vi "Event Loop Async.vi"(8 "error in (no error)":errorcluster, 11 "PanelArray in":refnum<class "PanelArray.lvclass">) -> ()   [LabVIEW 2018, in "OOPanel.lvlib" / "PanelArray.lvclass"]
uses:
  PanelArray.lvclass
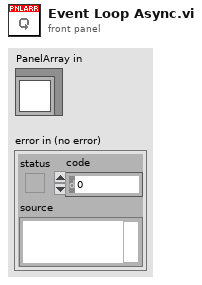
[diagram p1: front panel]
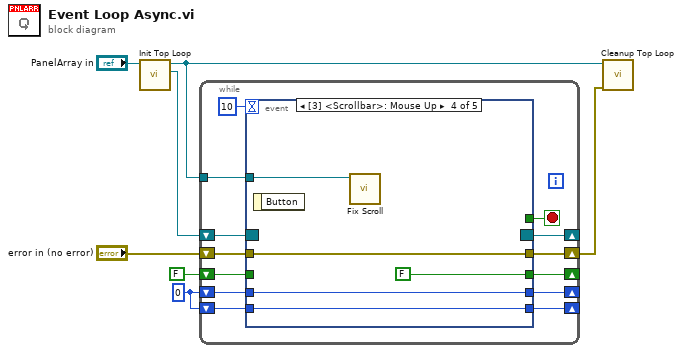
[diagram p0: block diagram]
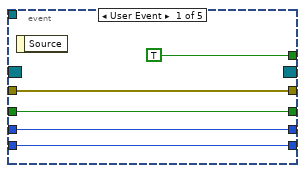
[diagram p2: hidden frame]
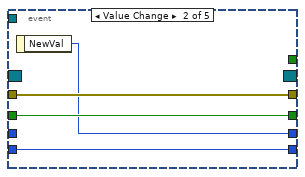
[diagram p3: hidden frame]
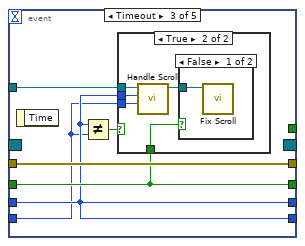
[diagram p4: hidden frame]
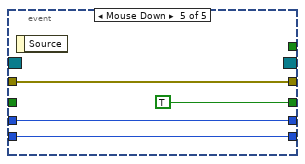
[diagram p7: hidden frame]
diagram:
  w1 = 0
  n1 = call "Init Top Loop.vi"("PanelArray in"="PanelArray in") -> ("Event Registration Refnum"=w6:refnum<event-registration>, "PanelArray out"=w4:refnum<class "PanelArray.lvclass">)  [unwired: 8 in, 1 out]
  n2 = while {
    tunnel: w4 -> [w19]
    shift-right: [w18] -> _
    shift-left: w6 -> [w20]
    shift-right: [w15] -> w3
    shift-left: "error in (no error)" -> [w16]
    shift-right: [w13] -> _
    shift-left: FALSE -> [w14]
    shift-right: [w9] -> _
    shift-left: w1 -> [w11]
    shift-right: [w8] -> _
    shift-left: w1 -> [w10]
    stop <- w17 stop-if-true
    n3 = event shown="[3] <Scrollbar>: Mouse Up" {
      selector: w20 -> [_ _ _ _ _]
      dyn-events: [_ _ _ _ _] -> w18
      timeout: 10 -> [_ _ _ _ _]
      tunnel: w19 -> [_ _ w34 w42 _]
      tunnel: [TRUE _ _ _ _] -> w17
      tunnel: w16 -> [w24 w29 w35 w46 w50]
      tunnel: [w24 w29 w35 w46 w50] -> w15
      tunnel: w14 -> [w23 w28 w33 _ _]
      tunnel: [w23 w28 w33 FALSE TRUE] -> w13
      tunnel: w11 -> [w21 _ w32 w43 w47]
      tunnel: w10 -> [w22 w26 w31 w44 w48]
      tunnel: [w21 w27 w32 w43 w47] -> w9
      tunnel: [w22 w26 w32 w44 w48] -> w8
      event User Event {
        n4 = event-data() -> ()  [unwired: 1 in, 1 out]
      }
      event Value Change {
        n5 = event-data() -> ("NewVal"=w27:i32)  [unwired: 1 in]
      }
      event Timeout {
        n6 = event-data() -> ()  [unwired: 1 in, 1 out]
        n7 = Not Equal?(x=w32, y=w31) -> (x != y?=w30:bool)
        n8 = case shown="True" w30 {
          tunnel: w34 -> [_ w40]
          tunnel: w32 -> [_ w39]
          tunnel: w31 -> [_ w38]
          tunnel: w33 -> [_ w37]
          frame False {
          }
          frame True {
            n9 = call "Handle Scroll.vi"("OldVal"=w38, "NewVal"=w39, "PanelArray in"=w40) -> ("PanelArray out"=w36:refnum<class "PanelArray.lvclass">)  [unwired: 7 in, 1 out]
            n10 = case shown="False" w37 {
              tunnel: w36 -> [w41 _]
              frame False {
                n11 = call "Fix Scroll.vi"("PanelArray in"=w41) -> ()  [unwired: 9 in, 2 out]
              }
              frame True {
              }
            }
          }
        }
      }
      event Mouse Up {
        n12 = event-data() -> ()  [unwired: 1 in, 1 out]
        n13 = call "Fix Scroll.vi"("PanelArray in"=w42) -> ()  [unwired: 9 in, 2 out]
      }
      event Mouse Down {
        n14 = event-data() -> ()  [unwired: 1 in, 1 out]
      }
    }
  }
  n15 = call "Cleanup Top Loop.vi"("error in (no error)"=w3, "PanelArray in"=w4) -> ()  [unwired: 8 in, 2 out]
